vi "Create Low Pass RC Filter (FGV).vi"(6 "fs (Hz)":dbl, 7 "init [F]":bool, 8 "error in (no error)":errorcluster, 9 "time constant (s)":dbl, 11 "stages":i32=2) -> (0 "error out":errorcluster, 3 "IIR Filters":T1(array[cluster]), 5 "init out":bool)   [LabVIEW 2019, in "DSP.lvclass"]
uses:
  DSP.lvclass
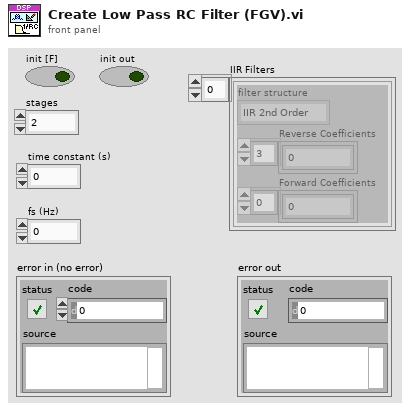
[diagram p1: front panel]
types:
  T1 = cluster{"filter structure":enum32{"IIR 2nd Order", "IIR 4th Order"}, "Reverse Coefficients":dbl[], "Forward Coefficients":dbl[]}[]
  T2 = cluster{"filter structure":enum32{"IIR 2nd Order", "IIR 4th Order"}, "Reverse Coefficients":dbl[], "Forward Coefficients":dbl[]}
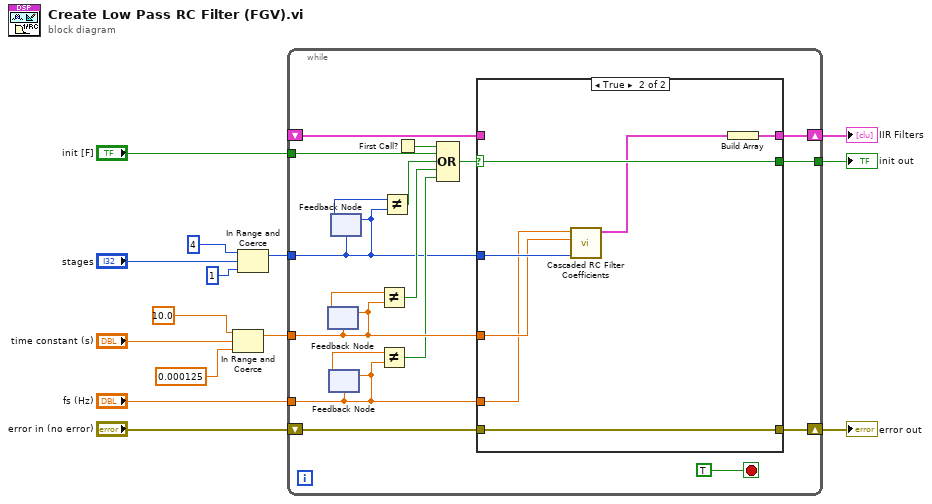
[diagram p0: block diagram]
diagram:
  n1 = In Range and Coerce(upper limit=10.0, x="time constant (s)", lower limit=0.000125) -> (coerced(x)=w1:dbl)  [unwired: 1 out]
  n2 = In Range and Coerce(upper limit=4, x="stages", lower limit=1) -> (coerced(x)=w2:i32)  [unwired: 1 out]
  n3 = while {
    tunnel: w1 -> [w21]
    tunnel: "fs (Hz)" -> [w24]
    shift-right: [w30] -> w14
    shift-left: "error in (no error)" -> [w31]
    shift-right: [w32] -> w4
    shift-left: _ -> [w27]
    tunnel: "init [F]" -> [w26]
    tunnel: w2 -> [w17]
    tunnel: [w15] -> w6
    stop <- TRUE stop-if-true
    n4 = feedback #1(w21) -> (w22:dbl)
    n5 = feedback-in #1(w21) -> ()
    n6 = feedback #2(w24) -> (w23:dbl)
    n7 = feedback-in #2(w24) -> ()
    n8 = feedback #3(w17) -> (w20:i32)
    n9 = feedback-in #3(w17) -> ()
    n10 = Not Equal?(x=w22, y=w21) -> (x != y?=w28:bool)
    n11 = Not Equal?(x=w23, y=w24) -> (x != y?=w19:bool)
    n12 = Not Equal?(x=w20, y=w17) -> (x != y?=w18:bool)
    n13 = First Call?() -> (First Call?: T/F=w16:bool)
    n14 = Compound Arithmetic op=OR(w16, w26, w18, w28, w19) -> (w25:bool)
    n15 = case shown="True" w25 {
      selector: w25 -> [w33 w42]
      tunnel: [w35 w40] -> w32
      tunnel: w31 -> [w34 w41]
      tunnel: [w34 w41] -> w30
      tunnel: w21 -> [_ w38]
      tunnel: w24 -> [_ w37]
      tunnel: w27 -> [w35 _]
      tunnel: w17 -> [_ w39]
      tunnel: [w33 w42] -> w15
      frame False {
      }
      frame True {
        n16 = call "Cascaded RC Filter Coefficients.vi"("filter order"=w39, "Time Constant"=w38, "Sample rate (Hz)"=w37) -> ("IIR Filter Cluster"=w36:T2)  [unwired: 6 in, 2 out]
        n17 = Build Array(w36) -> (w40:T1)
      }
    }
  }
  "init out" <- w6
  "IIR Filters" <- w4
  "error out" <- w14
